vi "Questão 1 - lista.vi"() -> ()   [LabVIEW 2019]
panel:
  out "Waveform Graph":dynamicdata(graph)
  in  "Phase":dbl[](array[numeric])
  in  "Amplitude":dbl[](array[numeric])
  in  "Frequency":dbl[](array[numeric])
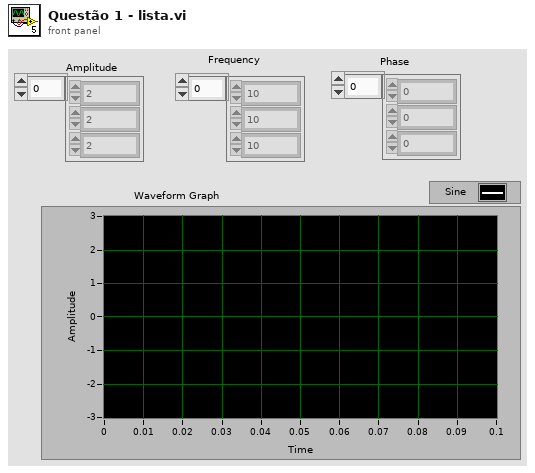
[diagram p1: front panel]
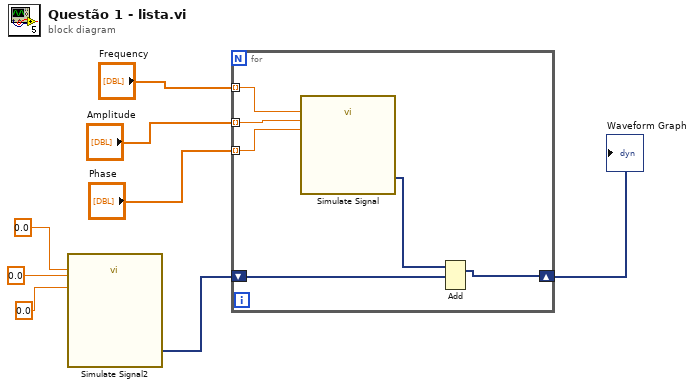
[diagram p0: block diagram]
diagram:
  n1 = call "Simulate Signal2"("Frequency"=0.0, "Amplitude"=0.0, "Phase"=0.0 ("Amplitude")) -> ("Sine"=w4:dynamicdata)  [unwired: 11 in, 1 out]
  n2 = for {
    shift-right: [w9] -> w5
    shift-left: w4 -> [w12]
    tunnel: "Frequency" -> [w11] mode=indexing
    tunnel: "Amplitude" -> [w14] mode=indexing
    tunnel: "Phase" -> [w13] mode=indexing
    n3 = call "Simulate Signal"("Frequency"=w11, "Amplitude"=w14, "Phase"=w13) -> ("Sine"=w10:dynamicdata)  [unwired: 11 in, 1 out]
    n4 = Add(1:w12, 2:w10) -> (0:w9:dynamicdata)  [unwired: 1 in, 1 out]
  }
  "Waveform Graph" <- w5
